vi "PC_Send_RS232.vi"() -> ()   [LabVIEW 2011]
uses:
  <vilib>/Instr/_visa.llb/VISA Configure Serial Port (Instr).vi
panel:
  in  "Send":bool
  in  "milliseconds to wait":u32=1000
  in  "Stop":bool
  in  "write buffer":string="Amtec"
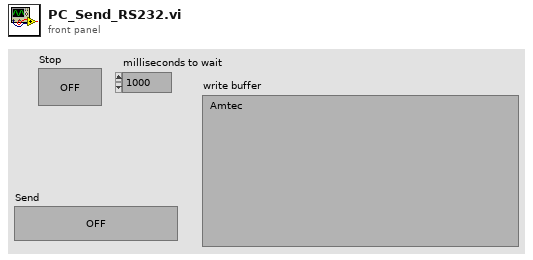
[diagram p1: front panel]
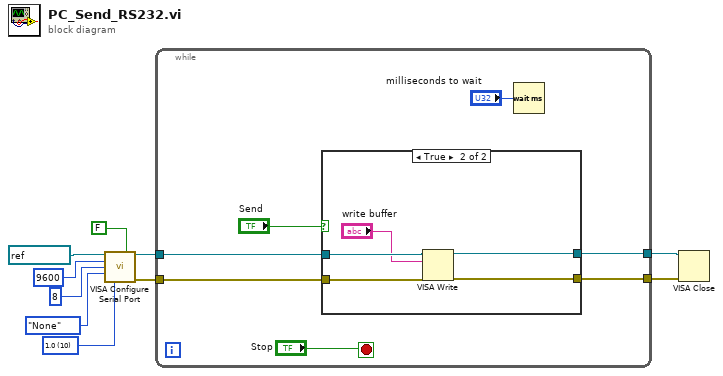
[diagram p0: block diagram]
diagram:
  w6 = u16 10 items=["1.0"=10, "1.5"=15, "2.0"=20] ("stop bits (10: 1 bit)")
  n1 = call-poly "VISA Configure Serial Port"("VISA resource name"=refnum<visa-resource-name> "COM6", "Enable Termination\nChar (T)"=FALSE ("Enable Termination\nChar (T)"), "baud rate (9600)"=u32 9600, "data bits (8)"=u16 8, "parity (0:none)"=enum16{"None", "Odd", "Even", "Mark", "Space"}."None", "stop bits (10: 1 bit)"=w6) -> ("VISA resource name out"=w4:refnum<visa-resource-name>, "error out"=w5:errorcluster)  [unwired: 8 in]
  n2 = while {
    tunnel: w5 -> [w17]
    tunnel: w4 -> [w16]
    tunnel: [w13] -> w3
    tunnel: [w15] -> w2
    stop <- "Stop" stop-if-true
    n3 = case shown="True" "Send" {
      tunnel: w17 -> [w18 w24]
      tunnel: w16 -> [w19 w23]
      tunnel: [w19 w21] -> w15
      tunnel: [w18 w20] -> w13
      frame False {
      }
      frame True {
        n4 = VISA Write(VISA resource name=w23, write buffer="write buffer", error in (no error)=w24) -> (VISA resource name out=w21:refnum<visa-resource-name>, error out=w20:errorcluster)  [unwired: 1 out]
      }
    }
    n5 = Wait (ms)(milliseconds to wait="milliseconds to wait") -> ()  [unwired: 1 out]
  }
  n6 = VISA Close(VISA resource name=w2, error in (no error)=w3) -> ()  [unwired: 1 out]
